vi "SMScriptTest.vi"() -> ()   [LabVIEW 2014, in "Bus_class.lvlib" / "Bus.lvclass"]
uses:
  Bus.lvclass
  <vilib>/Utility/config.llb/NI_LVConfig.lvlib
panel:
  out "Script 2":string[](array[string])
  in  "stop":bool
  in  "btnWrite":bool
  in  "btnRead":bool
  in  "Script":string[](array[string])=["foo,1,2,3", "bar", "doh", "ray"]
  in  "PathtoIniFile":path=path "D:/Projects/Framework/Events/EventPlugins/C37EvtPlugin/C37EventPlugin.ini"
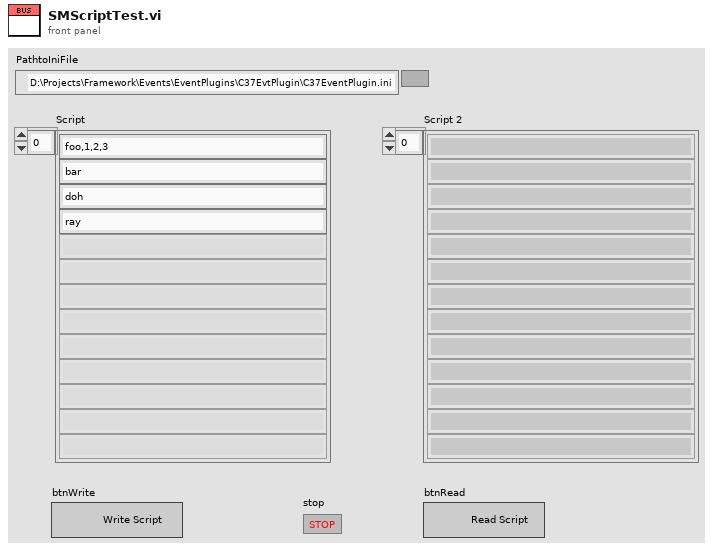
[diagram p1: front panel]
types:
  T1 = typedef "NI_LVConfig.lvlib/Config Data RefNum.ctl" = refnum<k1>
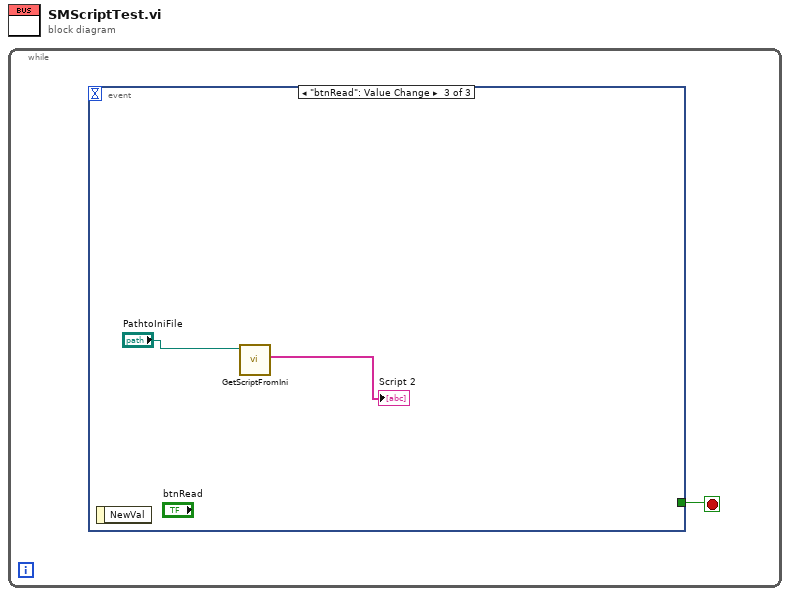
[diagram p0: block diagram]
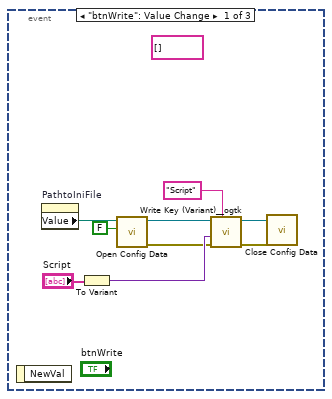
[diagram p2: hidden frame]
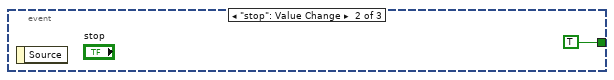
[diagram p3: hidden frame]
diagram:
  n1 = while {
    stop <- w1 stop-if-true
    n2 = event shown="[2] \"btnRead\": Value Change" {
      selector: _ -> [_ _ _]
      dyn-events: _ -> [_ _ _]
      timeout: _ -> [_ _ _]
      tunnel: [_ TRUE _] -> w1
      event "btnWrite": Value Change {
        (unwired) string[] []
        n3 = event-data() -> ()  [unwired: 1 in, 1 out]
        n4 = property on="PathtoIniFile" class="Path"() -> ("Value"=w10:path)  [unwired: 2 in, 2 out]
        n5 = To Variant(anything="Script") -> (Variant=w7:variant)
        n6 = call <vilib>:"Open Config Data.vi"("create file if necessary (T)"=FALSE, "configuration file path"=w10) -> ("error out"=w6:errorcluster, "refnum"=w5:T1)  [unwired: 7 in, 1 out]
        n7 = call <userlib>:"Write Key (Variant)__ogtk.vi"("section"="Script", "error in (no error)"=w6, "key-value"=w7, "refnum"=w5) -> ("error out"=w3:errorcluster, "refnum out"=w2:T1)  [unwired: 6 in]
        n8 = call <vilib>:"Close Config Data.vi"("error in (no error)"=w3, "refnum"=w2) -> ()  [unwired: 8 in, 2 out]
      }
      event "stop": Value Change {
        n9 = event-data() -> ()  [unwired: 1 in, 1 out]
      }
      event "btnRead": Value Change {
        n10 = event-data() -> ()  [unwired: 1 in, 1 out]
        n11 = call "GetScriptFromIni.vi"("PathtoIniFile"="PathtoIniFile") -> ("Script"=→"Script 2":string[])  [unwired: 9 in, 1 out]
      }
    }
  }
